vi "Set Node Attributes.vi"(8 "error in (no error)":errorcluster, 9 "values":string[](array[string]), 10 "names":string[](array[string]), 11 "node in":refnum<k20>) -> (0 "error out":errorcluster, 3 "node out":refnum<k20>)   [LabVIEW 2017, in "Error File Management.lvlib"]
uses:
  Error File Management.lvlib
  <vilib>/xml/Close Reference(Node).vi
  <vilib>/xml/Close Reference(NNMap).vi
  <resource>/objmgr/DOMUserDefRef.rc
  <vilib>/xml/NI_XML.lvlib
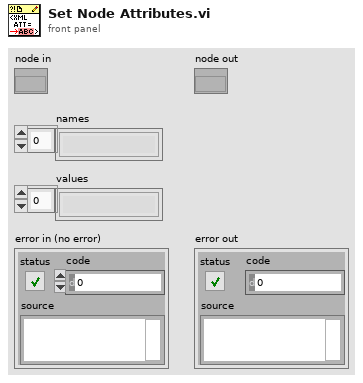
[diagram p1: front panel]
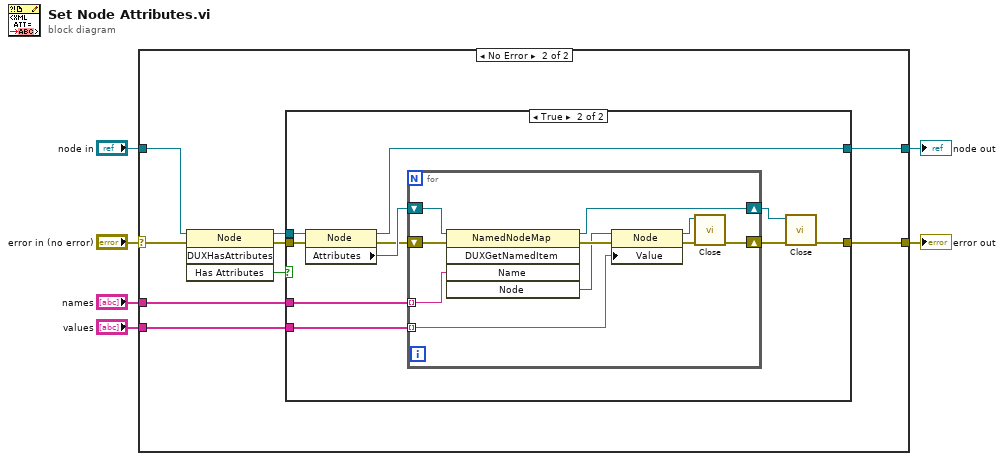
[diagram p0: block diagram]
diagram:
  n1 = case shown="No Error" "error in (no error)" {
    selector: "error in (no error)" -> [w8 w12]
    tunnel: "names" -> [_ w14]
    tunnel: [w8 w13] -> w4
    tunnel: "node in" -> [w7 w11]
    tunnel: [w7 w10] -> w2
    tunnel: "values" -> [_ w9]
    frame Error {
    }
    frame No Error {
      n2 = invoke class="Node" method="DUXHasAttributes"(reference=w11, error in=w12) -> (reference out=w17:refnum<k20>, error out=w16:errorcluster, "Has Attributes"=w15:bool)  [unwired: 2 in, 1 out]
      n3 = case shown="True" w15 {
        tunnel: w17 -> [w18 w28]
        tunnel: w16 -> [w19 w27]
        tunnel: w14 -> [_ w26]
        tunnel: [w19 w22] -> w13
        tunnel: [w18 w21] -> w10
        tunnel: w9 -> [_ w20]
        frame False {
        }
        frame True {
          n4 = property class="Node"(reference=w28, error in=w27) -> (reference out=w21:refnum<k20>, error out=w23:errorcluster, "Attributes"=w29:refnum<k20>)
          n5 = for {
            tunnel: w26 -> [w34] mode=indexing
            shift-right: [w33] -> w25
            shift-left: w23 -> [w32]
            shift-right: [w31] -> w24
            shift-left: w29 -> [w35]
            tunnel: w20 -> [w30] mode=indexing
            n6 = invoke class="NamedNodeMap" method="DUXGetNamedItem"(reference=w35, error in=w32, "Name"=w34) -> (reference out=w31:refnum<k20>, error out=w37:errorcluster, "Node"=w36:refnum<k20>)  [unwired: 2 in, 2 out]
            n7 = property class="Node"(reference=w36, error in=w37, "Value"=w30) -> (reference out=w39:refnum<k20>, error out=w38:errorcluster)
            n8 = call-poly <vilib>:"Close.vi"("error in (no error)"=w38, "node"=w39) -> ("error out"=w33:errorcluster)  [unwired: 7 out]
          }
          n9 = call-poly <vilib>:"Close.vi"("error in (no error)"=w25, "named node map"=w24) -> ("error out"=w22:errorcluster)  [unwired: 7 out]
        }
      }
    }
  }
  "error out" <- w4
  "node out" <- w2
